vi "File Page - Get Waveforms.vi"(8 "error in (no error)":errorcluster, 10 "File Waveforms in":T2 {"Node Refs" format="%.0x"}, 11 "Item Ref in":T1 format="%.0x") -> (0 "error out":errorcluster, 2 "File Waveforms out":T2 {"Node Refs" format="%.0x"}, 3 "Item Ref out":T1 format="%.0x")   [LabVIEW 2012, in "Waveform Data Logger System Explorer.lvlib"]
uses:
  Waveform Data Logger System Explorer.lvlib
  Types/File - Waveforms.ctl
  <vilib>/NI Veristand/Custom Device API/Custom Device Item Ref.ctl
  Shared/Globals/Property Strings.vi
  <vilib>/NI Veristand/Custom Device API/Get Item Property (String Array).vi
  <vilib>/NI Veristand/Custom Device API/Get Item Property (U32 Array).vi
  <vilib>/NI VeriStand/Custom Device API/Custom Device API.lvlib
  <vilib>/NI VeriStand/Custom Device Tools/Custom Device Utility Library/Custom Device Utility Library.lvlib
  Shared/Waveform Data Logger Shared.lvlib
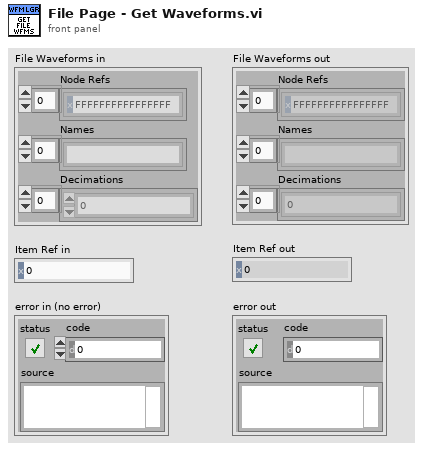
[diagram p1: front panel]
types:
  T1 = typedef "Custom Device API.lvlib/Custom Device Item Ref.ctl" = u64
  T2 = typedef "Waveform Data Logger System Explorer.lvlib/File - Waveforms.ctl" = cluster{"Node Refs":T1[], "Names":string[], "Decimations":u32[]}
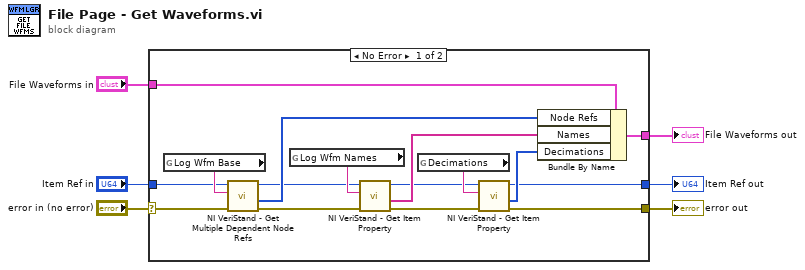
[diagram p0: block diagram]
diagram:
  n1 = case shown="No Error" "error in (no error)" {
    selector: "error in (no error)" -> [w7 w25]
    tunnel: [w22 w23] -> w6
    tunnel: "File Waveforms in" -> [w18 w23]
    tunnel: [w17 w25] -> w4
    tunnel: [w16 w24] -> w3
    tunnel: "Item Ref in" -> [w10 w24]
    frame No Error {
      n2 = global read "Property Strings.vi" "Log Wfm Base"() -> (w12:string)
      n3 = call <vilib>:"NI VeriStand - Get Multiple Dependent Node Refs.vi"("error in (no error)"=w7, "Base Property Name"=w12, "Item Ref in"=w10) -> ("error out"=w8:errorcluster, "Dependent Node Refs"=w19:T1[], "Item Ref out"=w9:T1)  [unwired: 6 in]
      n4 = global read "Property Strings.vi" "Log Wfm Names"() -> (w11:string)
      n5 = call-poly <vilib>:"NI VeriStand - Get Item Property.vi"("error in (no error)"=w8, "Property Name"=w11, "Item Ref in"=w9) -> ("error out"=w14:errorcluster, "Value"=w20:string[], "Item Ref out"=w13:T1)  [unwired: 1 in, 5 out]
      n6 = global read "Property Strings.vi" "Decimations"() -> (w15:string)
      n7 = call-poly <vilib>:"NI VeriStand - Get Item Property.vi"("error in (no error)"=w14, "Property Name"=w15, "Item Ref in"=w13) -> ("error out"=w17:errorcluster, "Value"=w21:u32[], "Item Ref out"=w16:T1)  [unwired: 1 in, 5 out]
      n8 = Bundle By Name(cluster=w18, "Node Refs"=w19, "Names"=w20, "Decimations"=w21) -> (w22:T2)
    }
    frame Error {
    }
  }
  "File Waveforms out" <- w6
  "error out" <- w4
  "Item Ref out" <- w3
